vi "Add State(s) to Queue By BOOL(Element).vi"(4 "False(Empty)":string, 6 "TRUE(Empty)":string, 8 "High Priority(FALSE)":bool, 10 "Bool":bool, 11 "Remaining States":string) -> (3 "States Out":string)   [LabVIEW 2014, in "JKI-State-Machine-Plus.lvlib"]
doc: "Depending on the High Priority and Bool input, this VI generates a concatenated state of TRUE/False and Remaning States. The High Priority input determines if the TRUE or False string concatenates before/after the remaining states. The Bool input determines whether TRUE or False string to be concatenated."
uses:
  JKI-State-Machine-Plus.lvlib
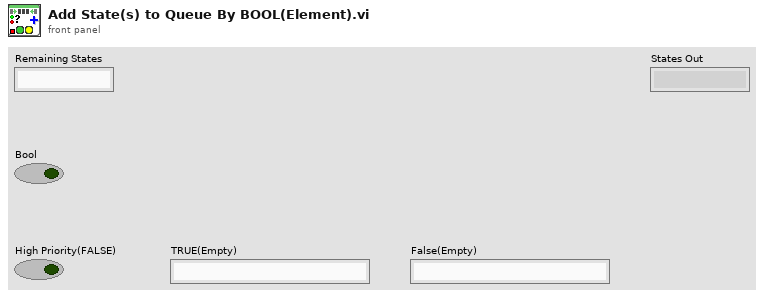
[diagram p1: front panel]
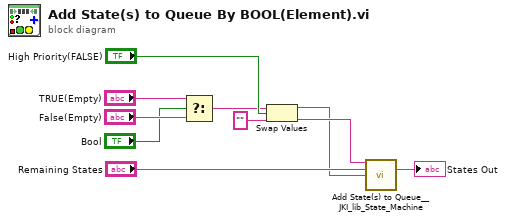
[diagram p0: block diagram]
diagram:
  n1 = Select(t="TRUE(Empty)", s="Bool", f="False(Empty)") -> (s? t:f=w4:string)
  n2 = Swap Values(12:w4, 13:"High Priority(FALSE)", 14:"") -> (1:w1:string, 3:w2:string)
  n3 = call <vilib>:"Add State(s) to Queue__JKI_lib_State_Machine.vi"("State(s) in Front (\"\")"=w2, "State(s) in (\"\")"="Remaining States", "State(s) at Back (\"\")"=w1) -> ("States Out"=→"States Out":string)  [unwired: 12 in]
